vi "weightExample_S.vi"(1 "weight":string) -> (0 "String":string="String")   [LabVIEW 2019]
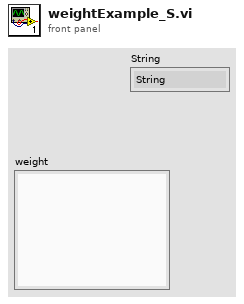
[diagram p1: front panel]
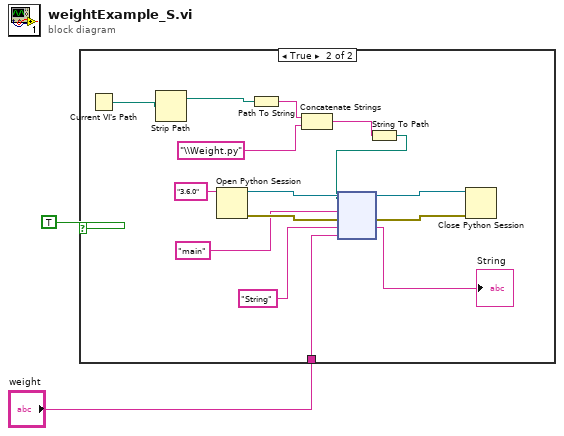
[diagram p0: block diagram]
diagram:
  n1 = case shown="True" TRUE {
    tunnel: "weight" -> [_ w11]
    frame False {
    }
    frame True {
      n2 = Current VI's Path() -> (path=w10:path)
      n3 = Strip Path(path=w10) -> (stripped path=w9:path)  [unwired: 1 out]
      n4 = Open Python Session(python version="3.6.0" ("Python version")) -> (session out=w17:refnum<k35>, error out=w16:errorcluster)  [unwired: 2 in]
      n5 = Path To String(path=w9) -> (string=w7:string)
      n6 = Concatenate Strings(w7, "\\Weight.py") -> (w6:string)
      n7 = String To Path(string=w6) -> (path=w5:path)
      n8 = node(w17, w5, "main" ("function name"), w16, "String", w11) -> (w14:refnum<k35>, w15:errorcluster, →"String":string)  [unwired: 1 in, 2 out]
      n9 = Close Python Session(session in=w14, error in=w15) -> ()  [unwired: 1 out]
    }
  }
